vi "Write Config File.vi"() -> ()   [LabVIEW 2019]
uses:
  RT Controls/Main Box Config.ctl
  RT Controls/FPGA State.ctl
  <vilib>/Utility/config.llb/Write Key (I32).vi
  <vilib>/Utility/config.llb/Write Key (Double).vi
  <vilib>/Utility/config.llb/Write Key (Boolean).vi
  <vilib>/Utility/config.llb/Write Key (U32).vi
  <vilib>/Utility/config.llb/Write Key (String).vi
  <vilib>/Utility/config.llb/NI_LVConfig.lvlib
panel:
  out "error out":errorcluster
  out "config path":path
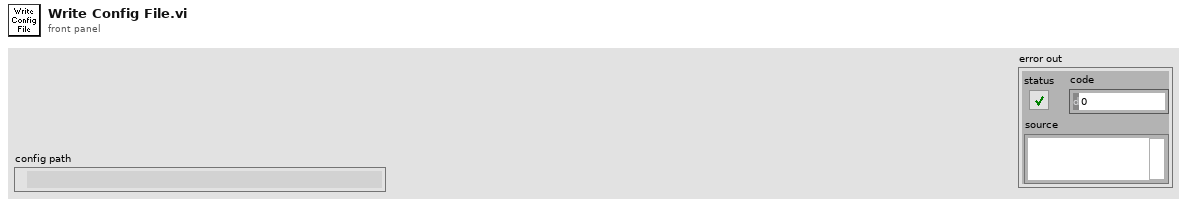
[diagram p1: front panel]
types:
  T1 = typedef "NI_LVConfig.lvlib/Config Data RefNum.ctl" = refnum<k1>
  T2 = typedef "FPGA State.ctl" = cluster{"mode request":enum16{"stop", "home", "position", "center"}, "az last rotation":enum16{"none", "forward", "reverse"}, "emergency stop":bool, "error?":bool, "errors":cluster{"emergency stop":bool, "encoder":bool, "az timeout":bool, "m1":bool, "m2":bool, "m4":bool}, "az enc counts":u64, "az pos":fxp<+/-,32,2>, "mode":u8, "sub mode":u8, "enc status":u16, "buttons":cluster{"em-stop":bool, "forward":bool, "reverse":bool, "open":bool, "close":bool, "up":bool, "down":bool, "force stop":bool}, "cloud?":bool, "cloud to counter":u32, "az to counter":u32, "env sensor":bool, "home sensor":bool, "rev dly counter":u32, "cmd request":i8, "cmd":i8, "config":cluster{"io.cloud-enable":bool, "io.encoder-negate":bool, "io.encoder-ref":u64, "io.encoder-step":u64, "io.home-pos":fxp<+/-,32,2>, "sm.az-timeout (ms)":u32, "sm.encoder-no-error":u16, "sm.main-pos-hs-thres":fxp<+/-,32,2>, "sm.main-pos-tol":fxp<+/-,32,2>, "sm.cloud-timeout (ms)":u32, "sm.rev-dly (ms)":u32, "io.encoder-center":u64, "sm-main-center-hs-thres":u64, "sm-main-center-tol":u64}, "homing?":bool, "homed?":bool, "az pos req":fxp<+/-,32,2>, "homing wait counter":u32, "config out":cluster{"io.cloud-enable":bool, "io.encoder-negate":bool, "io.encoder-ref":u64, "io.encoder-step":u64, "io.home-pos":fxp<+/-,32,2>, "sm.az-timeout (ms)":u32, "sm.encoder-no-error":u16, "sm.main-pos-hs-thres":fxp<+/-,32,2>, "sm.main-pos-tol":fxp<+/-,32,2>, "sm.cloud-timeout (ms)":u32, "sm.rev-dly (ms)":u32, "io.encoder-center":u64, "sm-main-center-hs-thres":u64, "sm-main-center-tol":u64}, "Chassis Temperature":i16}
  T3 = typedef "Main Box Config.ctl" = cluster{"WatchdogTim":i32, "DirRevDel":i32, "Coast":dbl, "HSThres":dbl, "EncCounts360":u64, "HomePos":dbl, "EncRefDeg":dbl, "EncRefCounts":u64, "Tol":dbl, "CloudEn":bool, "AutoShutEn":bool, "RainTim":i32, "AZTimeout":i32, "AZEncPol":enum16{"Positive", "Negative"}}
  T4 = cluster{"io.cloud-enable":bool, "io.encoder-negate":bool, "io.encoder-ref":u64, "io.encoder-step":u64, "io.home-pos":fxp<+/-,32,2>, "sm.az-timeout (ms)":u32, "sm.encoder-no-error":u16, "sm.main-pos-hs-thres":fxp<+/-,32,2>, "sm.main-pos-tol":fxp<+/-,32,2>, "sm.cloud-timeout (ms)":u32, "sm.rev-dly (ms)":u32, "io.encoder-center":u64, "sm-main-center-hs-thres":u64, "sm-main-center-tol":u64}
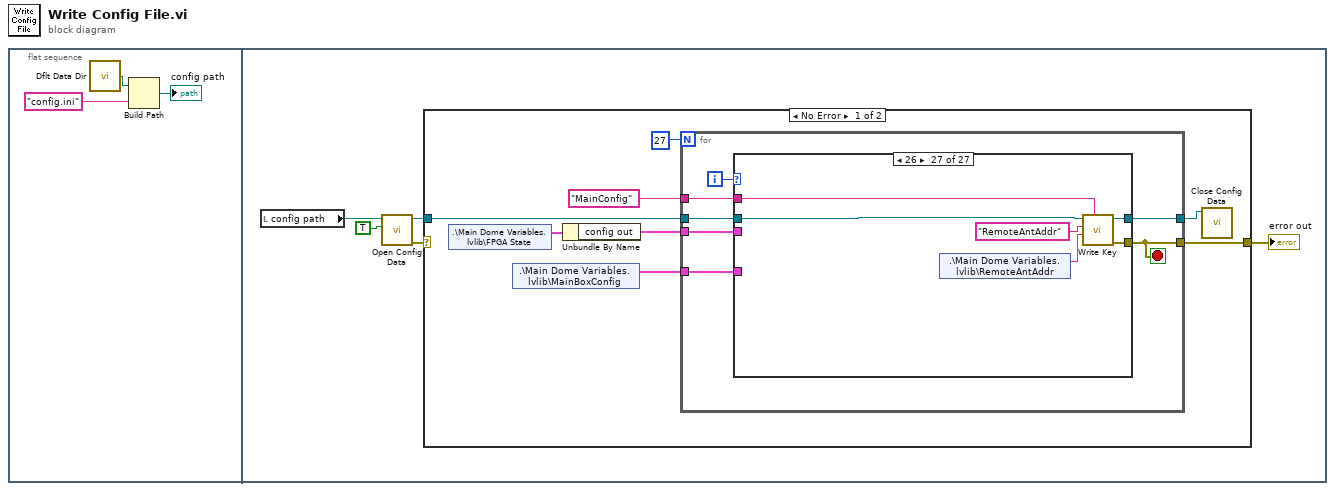
[diagram p0: block diagram]
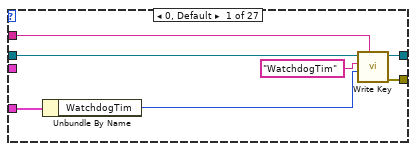
[diagram p2: hidden frame]
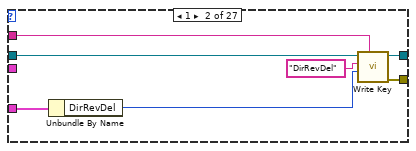
[diagram p3: hidden frame]
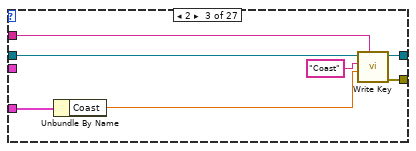
[diagram p4: hidden frame]
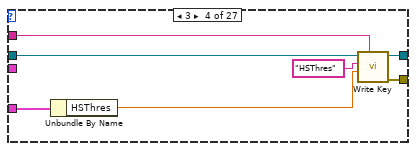
[diagram p5: hidden frame]
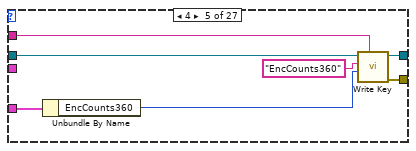
[diagram p6: hidden frame]
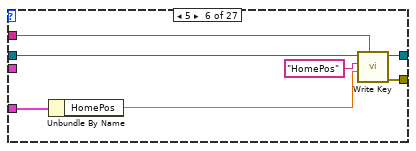
[diagram p7: hidden frame]
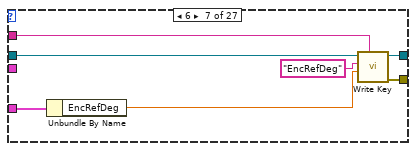
[diagram p8: hidden frame]
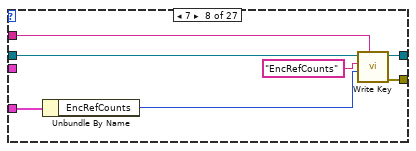
[diagram p9: hidden frame]
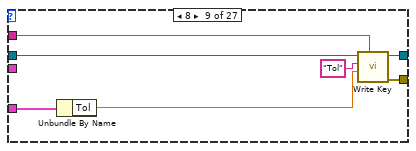
[diagram p10: hidden frame]
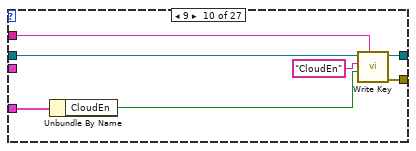
[diagram p11: hidden frame]
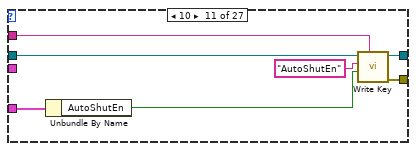
[diagram p12: hidden frame]
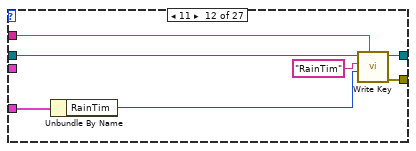
[diagram p13: hidden frame]
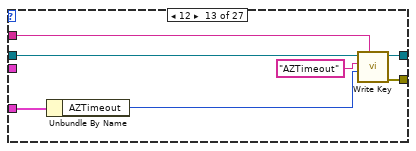
[diagram p14: hidden frame]
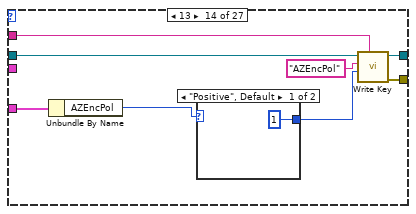
[diagram p15: hidden frame]
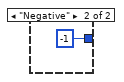
[diagram p16: hidden frame]
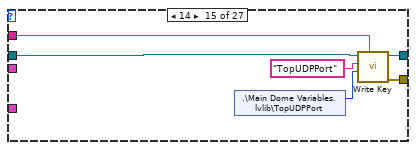
[diagram p17: hidden frame]
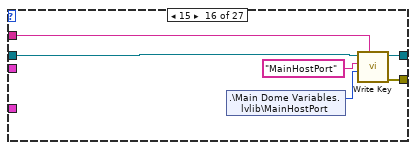
[diagram p18: hidden frame]
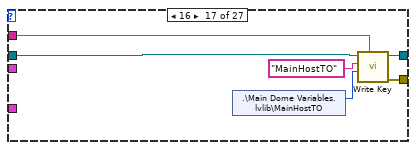
[diagram p19: hidden frame]
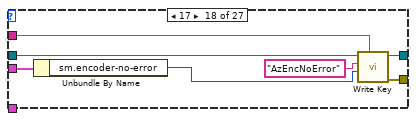
[diagram p20: hidden frame]
diagram:
  n1 = flat-sequence {
    frame #0 {
      n2 = call <vilib>:"Dflt Data Dir.vi"() -> ("App:Default Data Directory"=w3:path)
      n3 = Build Path(base path=w3, name or relative path="config.ini") -> (appended path=→"config path":path)
    }
    frame #1 {
      n4 = local read "config path"() -> (w6:path)
      n5 = call <vilib>:"Open Config Data.vi"("create file if necessary (T)"=TRUE, "configuration file path"=w6) -> ("error out"=w5:errorcluster, "refnum"=w7:T1)  [unwired: 7 in, 1 out]
      n6 = case shown="No Error" w5 {
        selector: w5 -> [_ w207]
        tunnel: w7 -> [w16 _]
        tunnel: [w12 w207] -> w4
        frame No Error {
          n7 = shared-variable ".\\Main Dome Variables.lvlib\\FPGA State"() -> (w10:T2)  [unwired: 1 in, 1 out]
          n8 = shared-variable ".\\Main Dome Variables.lvlib\\MainBoxConfig"() -> (w13:T3)  [unwired: 1 in, 1 out]
          n9 = Unbundle By Name(w10) -> ("config out"=w9:T4)
          n10 = for {
            N: 27 -> [_]
            tunnel: w16 -> [w21]
            tunnel: "MainConfig" ("section") -> [w22]
            tunnel: [w20] -> w14
            tunnel: w13 -> [w19]
            tunnel: [w18] -> w12
            tunnel: w9 -> [w17]
            i -> [w23]
            stop <- w18 stop-if-true
            n11 = case shown="26" w23 {
              tunnel: w22 -> [w30 w37 w44 w51 w58 w65 w72 w79 w86 w93 w100 w107 w114 w122 w129 w135 w141 w148 w155 w162 w169 w175 w181 w187 w193 w199 w205]
              tunnel: w21 -> [w29 w36 w43 w50 w57 w64 w71 w78 w85 w92 w99 w106 w113 w121 w130 w136 w142 w149 w156 w163 w170 w176 w182 w188 w194 w200 w206]
              tunnel: [w28 w35 w42 w49 w56 w63 w70 w77 w84 w91 w98 w105 w112 w120 w127 w133 w139 w146 w153 w160 w167 w173 w179 w185 w191 w197 w203] -> w20
              tunnel: w19 -> [w26 w33 w40 w47 w54 w61 w68 w75 w82 w89 w96 w103 w110 w118 _ _ _ _ _ _ _ _ _ _ _ _ _]
              tunnel: [w24 w31 w38 w45 w52 w59 w66 w73 w80 w87 w94 w101 w108 w115 w125 w131 w137 w145 w152 w159 w166 w172 w178 w184 w190 w196 w202] -> w18
              tunnel: w17 -> [_ _ _ _ _ _ _ _ _ _ _ _ _ _ _ _ _ w144 w151 w158 w164 _ _ _ _ _ _]
              frame 0, Default {
                n12 = Unbundle By Name(w26) -> ("WatchdogTim"=w25:i32)
                n13 = call-poly <vilib>:"Write Key.vi"("section"=w30, "value"=w25, "key"="WatchdogTim", "refnum"=w29) -> ("error out"=w24:errorcluster, "refnum out"=w28:T1)  [unwired: 5 in, 1 out]
              }
              frame 1 {
                n14 = Unbundle By Name(w33) -> ("DirRevDel"=w32:i32)
                n15 = call-poly <vilib>:"Write Key.vi"("section"=w37, "value"=w32, "key"="DirRevDel", "refnum"=w36) -> ("error out"=w31:errorcluster, "refnum out"=w35:T1)  [unwired: 5 in, 1 out]
              }
              frame 2 {
                n16 = Unbundle By Name(w40) -> ("Coast"=w39:dbl)
                n17 = call-poly <vilib>:"Write Key.vi"("section"=w44, "value"=w39, "key"="Coast", "refnum"=w43) -> ("error out"=w38:errorcluster, "refnum out"=w42:T1)  [unwired: 5 in, 1 out]
              }
              frame 3 {
                n18 = Unbundle By Name(w47) -> ("HSThres"=w46:dbl)
                n19 = call-poly <vilib>:"Write Key.vi"("section"=w51, "value"=w46, "key"="HSThres", "refnum"=w50) -> ("error out"=w45:errorcluster, "refnum out"=w49:T1)  [unwired: 5 in, 1 out]
              }
              frame 4 {
                n20 = Unbundle By Name(w54) -> ("EncCounts360"=w53:u64)
                n21 = call-poly <vilib>:"Write Key.vi"("section"=w58, "value"=w53, "key"="EncCounts360", "refnum"=w57) -> ("error out"=w52:errorcluster, "refnum out"=w56:T1)  [unwired: 5 in, 1 out]
              }
              frame 5 {
                n22 = Unbundle By Name(w61) -> ("HomePos"=w60:dbl)
                n23 = call-poly <vilib>:"Write Key.vi"("section"=w65, "value"=w60, "key"="HomePos", "refnum"=w64) -> ("error out"=w59:errorcluster, "refnum out"=w63:T1)  [unwired: 5 in, 1 out]
              }
              frame 6 {
                n24 = Unbundle By Name(w68) -> ("EncRefDeg"=w67:dbl)
                n25 = call-poly <vilib>:"Write Key.vi"("section"=w72, "value"=w67, "key"="EncRefDeg", "refnum"=w71) -> ("error out"=w66:errorcluster, "refnum out"=w70:T1)  [unwired: 5 in, 1 out]
              }
              frame 7 {
                n26 = Unbundle By Name(w75) -> ("EncRefCounts"=w74:u64)
                n27 = call-poly <vilib>:"Write Key.vi"("section"=w79, "value"=w74, "key"="EncRefCounts", "refnum"=w78) -> ("error out"=w73:errorcluster, "refnum out"=w77:T1)  [unwired: 5 in, 1 out]
              }
              frame 8 {
                n28 = Unbundle By Name(w82) -> ("Tol"=w81:dbl)
                n29 = call-poly <vilib>:"Write Key.vi"("section"=w86, "value"=w81, "key"="Tol", "refnum"=w85) -> ("error out"=w80:errorcluster, "refnum out"=w84:T1)  [unwired: 5 in, 1 out]
              }
              frame 9 {
                n30 = Unbundle By Name(w89) -> ("CloudEn"=w88:bool)
                n31 = call-poly <vilib>:"Write Key.vi"("section"=w93, "value"=w88, "key"="CloudEn", "refnum"=w92) -> ("error out"=w87:errorcluster, "refnum out"=w91:T1)  [unwired: 5 in, 1 out]
              }
              frame 10 {
                n32 = Unbundle By Name(w96) -> ("AutoShutEn"=w95:bool)
                n33 = call-poly <vilib>:"Write Key.vi"("section"=w100, "value"=w95, "key"="AutoShutEn", "refnum"=w99) -> ("error out"=w94:errorcluster, "refnum out"=w98:T1)  [unwired: 5 in, 1 out]
              }
              frame 11 {
                n34 = Unbundle By Name(w103) -> ("RainTim"=w102:i32)
                n35 = call-poly <vilib>:"Write Key.vi"("section"=w107, "value"=w102, "key"="RainTim", "refnum"=w106) -> ("error out"=w101:errorcluster, "refnum out"=w105:T1)  [unwired: 5 in, 1 out]
              }
              frame 12 {
                n36 = Unbundle By Name(w110) -> ("AZTimeout"=w109:i32)
                n37 = call-poly <vilib>:"Write Key.vi"("section"=w114, "value"=w109, "key"="AZTimeout", "refnum"=w113) -> ("error out"=w108:errorcluster, "refnum out"=w112:T1)  [unwired: 5 in, 1 out]
              }
              frame 13 {
                n38 = Unbundle By Name(w118) -> ("AZEncPol"=w117:enum16{"Positive", "Negative"})
                n39 = case shown="\"Positive\", Default" w117 {
                  tunnel: [1 -1] -> w116
                  frame "Positive", Default {
                  }
                  frame "Negative" {
                  }
                }
                n40 = call-poly <vilib>:"Write Key.vi"("section"=w122, "value"=w116, "key"="AZEncPol", "refnum"=w121) -> ("error out"=w115:errorcluster, "refnum out"=w120:T1)  [unwired: 5 in, 1 out]
              }
              frame 14 {
                n41 = shared-variable ".\\Main Dome Variables.lvlib\\TopUDPPort"() -> (w126:u16)  [unwired: 1 in, 1 out]
                n42 = call-poly <vilib>:"Write Key.vi"("section"=w129, "value"=w126, "key"="TopUDPPort", "refnum"=w130) -> ("error out"=w125:errorcluster, "refnum out"=w127:T1)  [unwired: 5 in, 1 out]
              }
              frame 15 {
                n43 = shared-variable ".\\Main Dome Variables.lvlib\\MainHostPort"() -> (w132:u16)  [unwired: 1 in, 1 out]
                n44 = call-poly <vilib>:"Write Key.vi"("section"=w135, "value"=w132, "key"="MainHostPort", "refnum"=w136) -> ("error out"=w131:errorcluster, "refnum out"=w133:T1)  [unwired: 5 in, 1 out]
              }
              frame 16 {
                n45 = shared-variable ".\\Main Dome Variables.lvlib\\MainHostTO"() -> (w138:u16)  [unwired: 1 in, 1 out]
                n46 = call-poly <vilib>:"Write Key.vi"("section"=w141, "value"=w138, "key"="MainHostTO", "refnum"=w142) -> ("error out"=w137:errorcluster, "refnum out"=w139:T1)  [unwired: 5 in, 1 out]
              }
              frame 17 {
                n47 = Unbundle By Name(w144) -> ("sm.encoder-no-error"=w143:u16)
                n48 = call-poly <vilib>:"Write Key.vi"("section"=w148, "value"=w143, "key"="AzEncNoError", "refnum"=w149) -> ("error out"=w145:errorcluster, "refnum out"=w146:T1)  [unwired: 5 in, 1 out]
              }
              frame 18 {
                n49 = Unbundle By Name(w151) -> ("io.encoder-center"=w150:u64)
                n50 = call-poly <vilib>:"Write Key.vi"("section"=w155, "value"=w150, "key"="EncCenter", "refnum"=w156) -> ("error out"=w152:errorcluster, "refnum out"=w153:T1)  [unwired: 5 in, 1 out]
              }
              frame 19 {
                n51 = Unbundle By Name(w158) -> ("sm-main-center-hs-thres"=w157:u64)
                n52 = call-poly <vilib>:"Write Key.vi"("section"=w162, "value"=w157, "key"="EncCenterHS", "refnum"=w163) -> ("error out"=w159:errorcluster, "refnum out"=w160:T1)  [unwired: 5 in, 1 out]
              }
              frame 20 {
                n53 = Unbundle By Name(w164) -> ("sm-main-center-tol"=w165:u64)
                n54 = call-poly <vilib>:"Write Key.vi"("section"=w169, "value"=w165, "key"="EncCenterTol", "refnum"=w170) -> ("error out"=w166:errorcluster, "refnum out"=w167:T1)  [unwired: 5 in, 1 out]
              }
              frame 21 {
                n55 = shared-variable ".\\Main Dome Variables.lvlib\\AntWifi"() -> (w171:bool)  [unwired: 1 in, 1 out]
                n56 = call-poly <vilib>:"Write Key.vi"("section"=w175, "value"=w171, "key"="AntWifi", "refnum"=w176) -> ("error out"=w172:errorcluster, "refnum out"=w173:T1)  [unwired: 5 in, 1 out]
              }
              frame 22 {
                n57 = shared-variable ".\\Main Dome Variables.lvlib\\TopAntAddr"() -> (w177:string)  [unwired: 1 in, 1 out]
                n58 = call-poly <vilib>:"Write Key.vi"("section"=w181, "value"=w177, "key"="TopAntAddr", "refnum"=w182) -> ("error out"=w178:errorcluster, "refnum out"=w179:T1)  [unwired: 5 in, 1 out]
              }
              frame 23 {
                n59 = shared-variable ".\\Main Dome Variables.lvlib\\TopAntPort"() -> (w183:u16)  [unwired: 1 in, 1 out]
                n60 = call-poly <vilib>:"Write Key.vi"("section"=w187, "value"=w183, "key"="TopAntPort", "refnum"=w188) -> ("error out"=w184:errorcluster, "refnum out"=w185:T1)  [unwired: 5 in, 1 out]
              }
              frame 24 {
                n61 = shared-variable ".\\Main Dome Variables.lvlib\\LocalAntAddr"() -> (w189:string)  [unwired: 1 in, 1 out]
                n62 = call-poly <vilib>:"Write Key.vi"("section"=w193, "value"=w189, "key"="LocalAntAddr", "refnum"=w194) -> ("error out"=w190:errorcluster, "refnum out"=w191:T1)  [unwired: 5 in, 1 out]
              }
              frame 25 {
                n63 = shared-variable ".\\Main Dome Variables.lvlib\\LocalAntSecret"() -> (w195:string)  [unwired: 1 in, 1 out]
                n64 = call-poly <vilib>:"Write Key.vi"("section"=w199, "value"=w195, "key"="LocalAntSecret", "refnum"=w200) -> ("error out"=w196:errorcluster, "refnum out"=w197:T1)  [unwired: 5 in, 1 out]
              }
              frame 26 {
                n65 = shared-variable ".\\Main Dome Variables.lvlib\\RemoteAntAddr"() -> (w201:string)  [unwired: 1 in, 1 out]
                n66 = call-poly <vilib>:"Write Key.vi"("section"=w205, "value"=w201, "key"="RemoteAntAddr", "refnum"=w206) -> ("error out"=w202:errorcluster, "refnum out"=w203:T1)  [unwired: 5 in, 1 out]
              }
            }
          }
          n67 = call <vilib>:"Close Config Data.vi"("refnum"=w14) -> ()  [unwired: 9 in, 2 out]
        }
        frame Error {
        }
      }
      "error out" <- w4
    }
  }
